vi "Set Search Results.vi"(6 "Search results":i32[](array[numeric]), 8 "error in (no error)":errorcluster, 11 "Composite Object in":refnum<class "CConfig Object.lvclass">) -> (0 "error out":errorcluster, 3 "Composite Object out":refnum<class "CConfig Object.lvclass">)   [LabVIEW 2013, in "CConfig Object.lvclass"]
doc: "Copyright 2018, Carya Automatisering, Wiebe Walstra."
uses:
  CConfig Object.lvclass
  CConfig Object.lvclass/CConfig Object.ctl
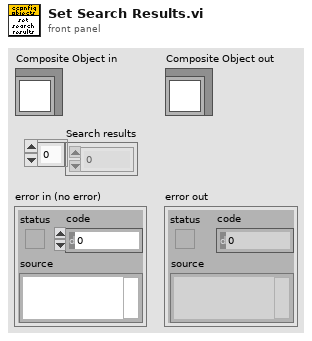
[diagram p1: front panel]
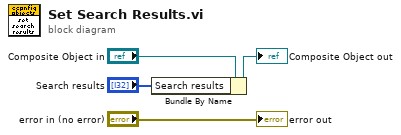
[diagram p0: block diagram]
diagram:
  n1 = Bundle By Name(cluster="Composite Object in", "Search results"="Search results") -> (→"Composite Object out":refnum<class "CConfig Object.lvclass">)
  "error out" <- "error in (no error)"
